vi "executeDefendAreaSkill.vi"(6 "Number of Defenders\nWithout Duelist":i32, 8 "error in (no error)":errorcluster, 9 "Robot in":refnum<class "Robot.lvclass">, 10 "Game":refnum<class "Game.lvclass">, 11 "DefendAreaSkill in":refnum<class "DefendAreaSkill.lvclass">) -> (0 "error out":errorcluster, 2 "Robot out":refnum<class "Robot.lvclass">, 3 "DefendAreaSkill out":refnum<class "DefendAreaSkill.lvclass">)   [LabVIEW 2023, in "DefendAreaSkill.lvclass"]
uses:
  DefendAreaSkill.lvclass
  Game_class/Game.lvclass
  Robot_class/Robot.lvclass
  Utilities_class/Utilities.lvclass
  Team_class/DefensivePlay.ctl
  Game_class/Game.lvclass/Game.ctl
  Parameters_class/Parameters.lvclass/Parameters.ctl
  Team_class/Team.lvclass/Team.ctl
  Robot_class/Robot.lvclass/Robot.ctl
  Game_class/Read BallRef.vi
  Game_class/Read Parameters.lvclass.vi
  Game_class/Read DefensiveTeam.vi
  Team_class/Read RobotRef.vi
  Team_class/Read DefensivePlay.vi
  Parameters_class/Read Area.vi
  Robot_class/Write dest_x.vi
  Robot_class/Write dest_y.vi
  Robot_class/Write dest_orientation.vi
  Ally_class/Ally.lvclass
  C:/Users/roboi/Downloads/VSS_AI-Larc2023 - Copia (2)/Team_class/Team.lvclass
  Ball_class/Ball.lvclass
  Parameters_class/Parameters.lvclass
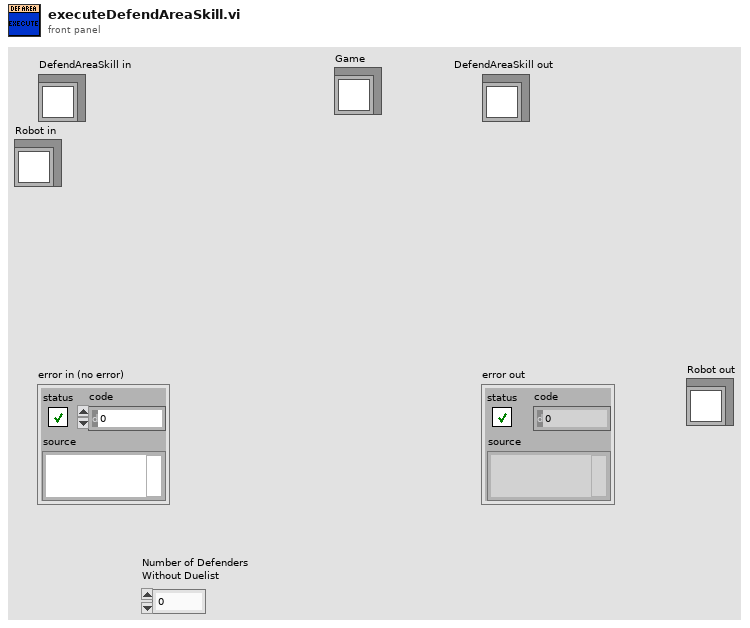
[diagram p1: front panel]
types:
  T1 = typedef "DefensivePlay.ctl" = enum16{"NormalDefensiveWithDuelist", "NormalDefensive", "TestPlay", "Halt", "Timeout", "PenaltyEnemy", "PenaltyAlly"}
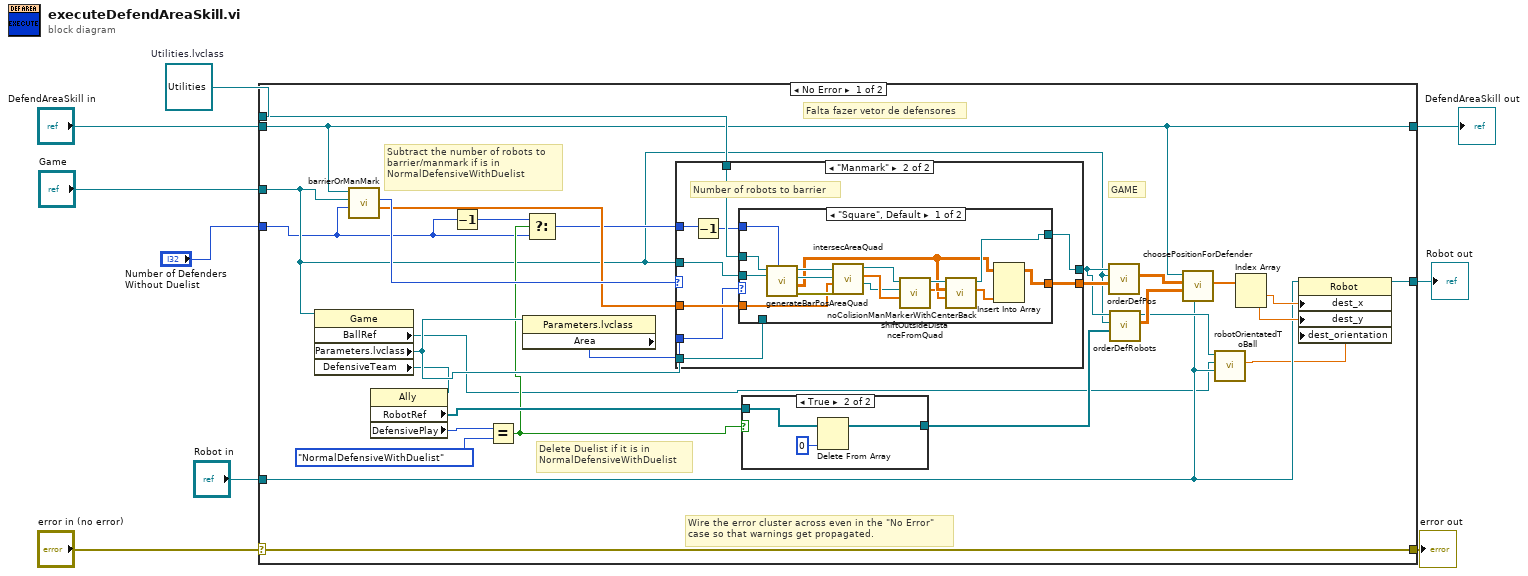
[diagram p0: block diagram]
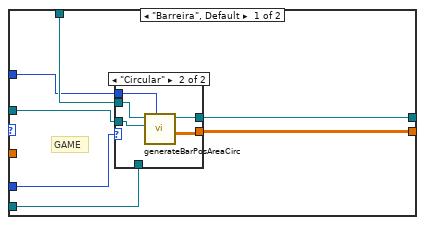
[diagram p3: hidden frame]
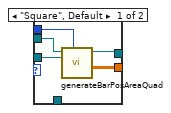
[diagram p4: hidden frame]
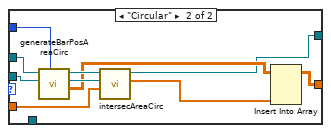
[diagram p5: hidden frame]
diagram:
  w4 = refnum<class "Utilities.lvclass"> refnum  # Utilities.lvclass
  n1 = case shown="No Error" "error in (no error)" {
    selector: "error in (no error)" -> [w38 w97]
    tunnel: [w38 w97] -> w8
    tunnel: [w32 w96] -> w6
    tunnel: "DefendAreaSkill in" -> [w32 w96]
    tunnel: "Game" -> [w12 _]
    tunnel: w4 -> [w36 _]
    tunnel: "Robot in" -> [w25 w95]
    tunnel: [w23 w95] -> w2
    tunnel: "Number of Defenders\nWithout Duelist" -> [w11 _]
    frame No Error {
      # "GAME"
      # "Subtract the number of robots to\nbarrier/manmark if is in\nNormalDefensiveWithDuelist"
      # "Delete Duelist if it is in\nNormalDefensiveWithDuelist"
      # "Falta fazer vetor de defensores"
      # "Wire the error cluster across even in the \"No Error\"\ncase so that warnings get propagated."
      n2 = property class="Game"(reference=w12) -> ("BallRef"=w10:refnum<class "Ball.lvclass">, "Parameters.lvclass"=w22:refnum<class "Parameters.lvclass">, "DefensiveTeam"=w20:refnum<class "Ally.lvclass">)  [unwired: 1 in, 2 out]
      n3 = call "barrierOrManMark.vi"("Number of Defenders\nWithout Duelist"=w11, "Game"=w12, "DefendAreaSkill in"=w32) -> ("Enemy position\nto mark"=w33:dbl[], "Type of Defense Barrier"=w37:enum16{"Barreira", "Manmark"})  [unwired: 5 in, 2 out]
      n4 = property class="Ally"(reference=w20) -> ("RobotRef"=w16:refnum<class "Robot.lvclass">[], "DefensivePlay"=w19:T1)  [unwired: 1 in, 2 out]
      n5 = Decrement(x=w11) -> (x-1=w14:i32)
      n6 = Equal?(x=w19, y=DefensivePlay."NormalDefensiveWithDuelist") -> (x = y?=w15:bool)
      n7 = property class="Parameters.lvclass"(reference=w22) -> ("Area"=w21:enum16{"Circular", "Square"})  [unwired: 1 in, 2 out]
      n8 = Select(t=w14, s=w15, f=w11) -> (s? t:f=w13:i32)
      n9 = case shown="\"Manmark\"" w37 {
        tunnel: w21 -> [w49 w62]
        tunnel: w36 -> [w48 w66]
        tunnel: w22 -> [w47 w68]
        tunnel: w12 -> [w46 w67]
        tunnel: [w45 w64] -> w35
        tunnel: [w44 w63] -> w34
        tunnel: w33 -> [_ w65]
        tunnel: w13 -> [w43 w61]
        frame "Barreira", Default {
          # "GAME"
          n10 = case shown="\"Circular\"" w49 {
            tunnel: w48 -> [w54 w59]
            tunnel: w47 -> [_ _]
            tunnel: w46 -> [w53 w58]
            tunnel: [w52 w57] -> w44
            tunnel: [w51 w56] -> w45
            tunnel: w43 -> [w50 w55]
            frame "Square", Default {
              n11 = call "generateBarPosAreaQuad.vi"("Number of Defenders\nWithout Duelist"=w50, "Game"=w53, "Utilities in"=w54) -> ("Pos Centers Back"=w51:dbl[][], "Utilities out"=w52:refnum<class "Utilities.lvclass">)  [unwired: 5 in, 2 out]
            }
            frame "Circular" {
              n12 = call "generateBarPosAreaCirc.vi"("Number of Denfenders\nWhithout Duelist"=w55, "Game"=w58, "Utilities in"=w59) -> ("Posição dos Defensores"=w56:dbl[][], "Utilities out"=w57:refnum<class "Utilities.lvclass">)  [unwired: 5 in, 2 out]
            }
          }
        }
        frame "Manmark" {
          # "Number of robots to barrier"
          n13 = Decrement(x=w61) -> (x-1=w60:i32)
          n14 = case shown="\"Square\", Default" w62 {
            tunnel: w66 -> [w84 w94]
            tunnel: w68 -> [_ _]
            tunnel: w67 -> [w83 w93]
            tunnel: w65 -> [w79 w90]
            tunnel: [w78 w87] -> w64
            tunnel: [w72 w86] -> w63
            tunnel: w60 -> [w77 w85]
            frame "Square", Default {
              n15 = call "generateBarPosAreaQuad.vi"("Number of Defenders\nWithout Duelist"=w77, "Game"=w83, "Utilities in"=w84) -> ("error out"=w82:errorcluster, "Pos Centers Back"=w71:dbl[][], "Game out"=w80:refnum<class "Game.lvclass">, "Utilities out"=w81:refnum<class "Utilities.lvclass">)  [unwired: 5 in]
              n16 = call "intersecAreaQuad.vi"("error in (no error)"=w82, "Ball/Enemy\nPosition"=w79, "Game"=w80, "Utilities in"=w81) -> ("Game"=w74:refnum<class "Game.lvclass">, "Pos de Interseção"=w76:dbl[], "Utilities out"=w75:refnum<class "Utilities.lvclass">)  [unwired: 4 in, 1 out]
              n17 = call "shiftOutsideDistanceFromQuad.vi"("Pos de Interseção"=w76, "Game"=w74, "Utilities in"=w75) -> ("Array"=w70:dbl[], "Utilities out"=w73:refnum<class "Utilities.lvclass">)  [unwired: 6 in, 1 out]
              n18 = call "noColisionManMarkerWithCenterBack.vi"("Pos ManMarker 2"=w70, "Pos CenterBacks"=w71, "Utilities in"=w73) -> ("Pos ManMarker"=w69:dbl[], "Utilities out"=w72:refnum<class "Utilities.lvclass">)  [unwired: 6 in, 1 out]
              n19 = Insert Into Array(array=w71, new element=w69) -> (w78:dbl[][])  [unwired: 2 in]
            }
            frame "Circular" {
              n20 = call "generateBarPosAreaCirc.vi"("Number of Denfenders\nWhithout Duelist"=w85, "Game"=w93, "Utilities in"=w94) -> ("Posição dos Defensores"=w89:dbl[][], "Game out"=w91:refnum<class "Game.lvclass">, "Utilities out"=w92:refnum<class "Utilities.lvclass">)  [unwired: 5 in, 1 out]
              n21 = call "intersecAreaCirc.vi"("Ball/Enemy\nPosition"=w90, "Game"=w91, "Utilities in"=w92) -> ("Position"=w88:dbl[], "Utilities out"=w86:refnum<class "Utilities.lvclass">)  [unwired: 6 in, 1 out]
              n22 = Insert Into Array(array=w89, new element=w88) -> (w87:dbl[][])  [unwired: 2 in]
            }
          }
        }
      }
      n23 = case shown="True" w15 {
        tunnel: [w39 w42] -> w17
        tunnel: w16 -> [w39 w41]
        frame False {
        }
        frame True {
          n24 = Delete From Array(array=w41, index=0) -> (array with subset deleted=w42:refnum<class "Robot.lvclass">[])  [unwired: 1 in, 1 out]
        }
      }
      n25 = call "orderDefPos.vi"("Def Positions"=w35, "Game"=w12, "Utilities in"=w34) -> ("Ordered Positions"=w31:dbl[][])  [unwired: 6 in, 2 out]
      n26 = call "orderDefRobots.vi"("Array of Robots"=w17, "Game"=w12, "Utilities in"=w34) -> ("Odered array of robots"=w30:dbl[][], "Utilities out"=w26:refnum<class "Utilities.lvclass">)  [unwired: 6 in, 1 out]
      n27 = call "choosePositionForDefender.vi"("Robot"=w25, "Odered array of robots"=w30, "Ordered Positions To Go"=w31, "DefendAreaSkill in"=w32) -> ("Position"=w29:dbl[])  [unwired: 5 in, 2 out]
      n28 = call "robotOrientatedToBall.vi"("Robot"=w25, "BallRef"=w10, "Utilities in"=w26) -> ("Orientation"=w24:dbl)  [unwired: 6 in, 2 out]
      n29 = Index Array(array=w29) -> (element #1=w28:dbl, element #2=w27:dbl)  [unwired: 2 in]
      n30 = property class="Robot"(reference=w25, "dest_x"=w28, "dest_y"=w27, "dest_orientation"=w24) -> (reference out=w23:refnum<class "Robot.lvclass">)  [unwired: 1 in, 1 out]
    }
    frame Error {
    }
  }
  "error out" <- w8
  "DefendAreaSkill out" <- w6
  "Robot out" <- w2
